vi "Init Comms.vi"(8 "error in (no error)":errorcluster, 11 "Communications in":refnum<class "Communications.lvclass">) -> (0 "error out":errorcluster, 3 "Communications out":refnum<class "Communications.lvclass">)   [LabVIEW 2021, in "Communications.lvclass"]
uses:
  Communications.lvclass
  C:/Program Files/National Instruments/LabVIEW 2021/vi.lib/ActorFramework/Actor/Actor.lvclass
  Publish-Subscribe/Context.ctl
  Communications.lvclass/Communications.ctl
  <vilib>/ActorFramework/Actor/Actor.lvclass/Actor.ctl
  <vilib>/ActorFramework/Message Enqueuer/Message Enqueuer.lvclass/Message Enqueuer.ctl
  Publish-Subscribe/Interfaces/Publisher Messages/Subscribe Msg/Subscribe Msg.lvclass/Subscribe Msg.ctl
  Read Communications Configuration.vi
  <vilib>/ActorFramework/Message Enqueuer/Init from Existing Queue.vi
  <vilib>/ActorFramework/Message Enqueuer/Enqueue.vi
  Publish-Subscribe/Interfaces/Publisher Messages/Subscribe Msg/Subscribe Msg.lvclass
  C:/Program Files/National Instruments/LabVIEW 2021/vi.lib/ActorFramework/Message/Message.lvclass
  <vilib>/ActorFramework/Message Priority Queue/Priority Enqueue.vi
  <vilib>/ActorFramework/Message Enqueuer/Message Enqueuer.lvclass
  <vilib>/ActorFramework/Actor/Actor.lvclass
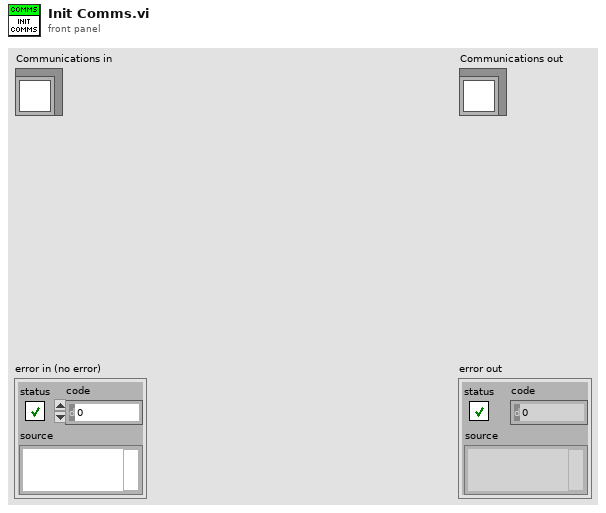
[diagram p1: front panel]
types:
  T1 = typedef "Context.ctl" = cluster{"Topic":string, "Source":string}
  T2 = typedef "Communications Configuration.ctl" = cluster{"Subscribe to modules":string[]}
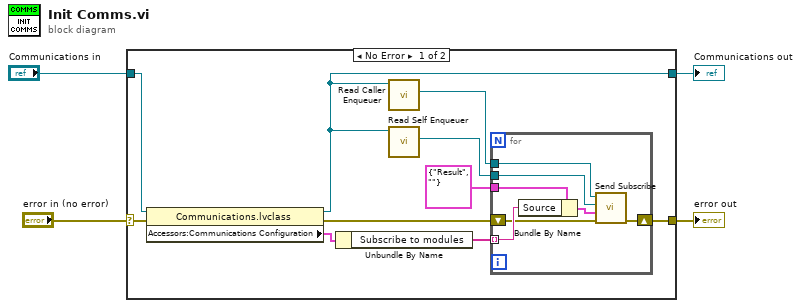
[diagram p0: block diagram]
diagram:
  n1 = case shown="No Error" "error in (no error)" {
    selector: "error in (no error)" -> [w14 w23]
    tunnel: [w9 w23] -> w3
    tunnel: [w8 w22] -> w1
    tunnel: "Communications in" -> [w13 w22]
    frame No Error {
      n2 = property class="Communications.lvclass"(reference=w13, error in=w14) -> (reference out=w8:refnum<class "Communications.lvclass">, error out=w10:errorcluster, "Accessors:Communications Configuration"=w12:T2)
      n3 = Unbundle By Name(w12) -> ("Subscribe to modules"=w11:string[])
      n4 = call <vilib>:"Read Caller Enqueuer.vi"("Actor"=w8) -> ("Caller Enqueuer"=w5:refnum<class "Message Enqueuer.lvclass">)  [unwired: 10 in]
      n5 = call <vilib>:"Read Self Enqueuer.vi"("Actor"=w8) -> ("Self Enqueuer"=w7:refnum<class "Message Enqueuer.lvclass">)  [unwired: 10 in]
      n6 = for {
        tunnel: w11 -> [w20] mode=indexing
        tunnel: w5 -> [w18]
        shift-right: [w15] -> w9
        shift-left: w10 -> [w19]
        tunnel: w7 -> [w17]
        tunnel: T1 {"Topic"="Result", "Source"=""} ("Context") -> [w21]
        n7 = Bundle By Name(cluster=w21, "Source"=w20) -> (w16:T1)
        n8 = call "Send Subscribe.vi"("error in (no error)"=w19, "Context"=w16, "Subscriber Enq"=w17, "Message Enqueuer"=w18) -> ("error out"=w15:errorcluster)  [unwired: 6 in, 1 out]
      }
    }
    frame Error {
    }
  }
  "error out" <- w3
  "Communications out" <- w1
